vi "Adquisicion.vi"(5 "Stop (F)":bool) -> (20 "Image Out":T1(plugin-control), 26 "Stopped":bool, 27 "error out":errorcluster)   [LabVIEW 2017]
doc: "Creates, and edits acquisitions using the NI Vision Acquisition Express VI.\n\nThe NI Vision Acquisition Wizard is launched by placing the Express VI on the block diagram. Select an acquisition source and configure an acquisition using NI-IMAQ, NI-IMAQdx, or simulate an acquisition by reading an AVI or image files from a folder. After an acquisition is configured, select controls and indicators to be able to programmatically set in LabVIEW. Double-click the Vision Acquisition Express VI to edit the acquisition.\n\nNote: Any images created by the Express VI need to be disposed after use. Use the IMAQ Dispose.vi to cleanup the images output by the Express VI when they are no longer needed."
uses:
  <vilib>/vision/driver/NI_Vision_Acquisition_Software.lvlib
  <vilib>/vision/driver/Vision Acquisition Express Utility VIs.llb/Vision Acquisition Path Convert (String).vi
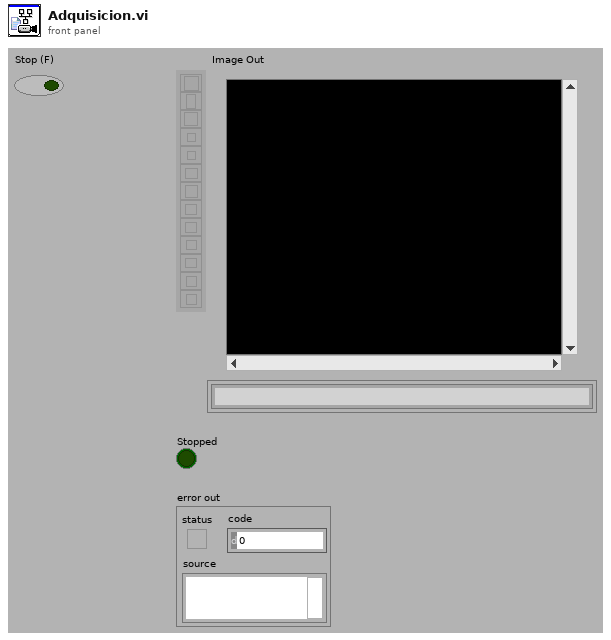
[diagram p1: front panel]
types:
  T1 = typedef "IMAQ Image.ctl" = refnum<image>
  T2 = typedef "IMAQdx.ctl" = refnum<k21>
  T3 = cluster{"File Type":string, "Quality":u32, "Compress":bool, "Lossless":bool, "Ratio":sgl, "Codec":string, "Frame Rate":u32, "Limit Frames":bool, "Max Frames":u32}
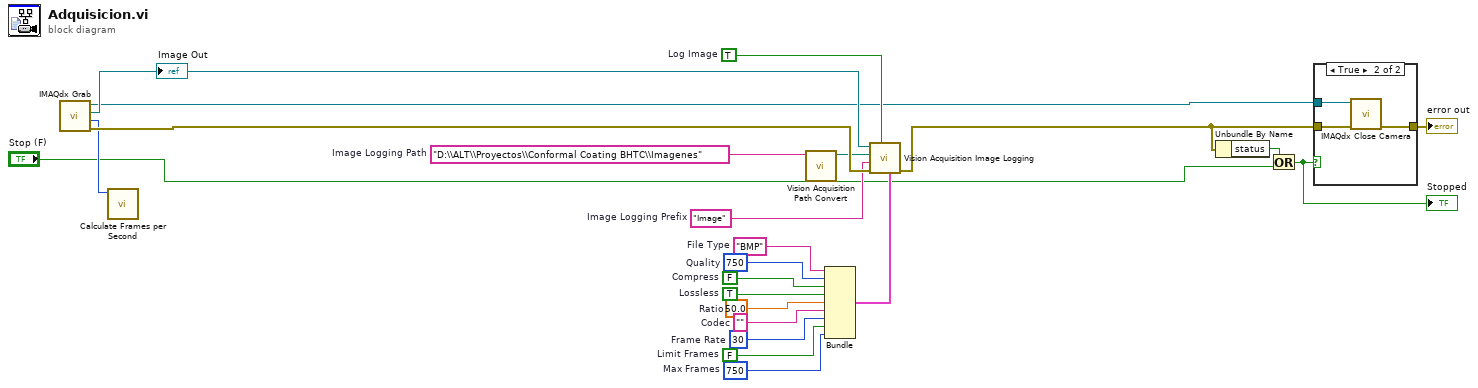
[diagram p0: block diagram]
diagram:
  w6 = "D:\\ALT\\Proyectos\\Conformal Coating BHTC\\Imagenes"  # Image Logging Path
  w9 = TRUE  # Log Image
  w20 = "Image"  # Image Logging Prefix
  w15 = sgl 50.0  # Ratio
  w16 = TRUE  # Lossless
  w17 = FALSE  # Compress
  w18 = u32 750  # Quality
  w14 = ""  # Codec
  w13 = u32 30  # Frame Rate
  w11 = u32 750  # Max Frames
  w12 = FALSE  # Limit Frames
  w19 = "BMP"  # File Type
  n1 = call <vilib>:"IMAQdx Grab.vi"() -> ("error out"=w23:errorcluster, "Buffer Number Out"=w22:u32, "Image Out"=w21:T1, "Session Out"=w5:T2, "error in"=w26:errorcluster, "Image In"=w25:T1, "Session In"=w24:T2)  [unwired: 1 in, 4 out]
  "Image Out" <- w21
  n2 = call <vilib>:"Calculate Frames per Second.vi"("Buffer Number"=w22) -> ()  [unwired: 2 in, 9 out]
  n3 = call-poly <vilib>:"Vision Acquisition Path Convert.vi"("Path In"=w6) -> ("Path Out"=w7:path)  [unwired: 10 in]
  n4 = Bundle("File Type"=w19, "Quality"=w18, "Compress"=w17, "Lossless"=w16, "Ratio"=w15, "Codec"=w14, "Frame Rate"=w13, "Limit Frames"=w12, "Max Frames"=w11) -> (w8:T3)  [unwired: 1 out]
  n5 = call <vilib>:"Vision Acquisition Image Logging.vi"("File Settings"=w8, "Log Image"=w9, "error in (no error)"=w23, "Image Logging Prefix"=w20, "Image Logging Path"=w7, "Image In"=w21) -> ("error out"=w10:errorcluster)  [unwired: 1 in, 4 out]
  n6 = Unbundle By Name(w10) -> ("status"=w1:bool)
  n7 = Or(x=w1, y="Stop (F)") -> (x .or. y?=w2:bool)
  "Stopped" <- w2
  n8 = case "Case Structure_template1" shown="True" w2 {
    tunnel: [w27 w29] -> w4
    tunnel: w10 -> [w27 w30]
    tunnel: w5 -> [_ w28]
    frame False {
    }
    frame True {
      n9 = call <vilib>:"IMAQdx Close Camera.vi"("error in"=w30, "Session In"=w28) -> ("error out"=w29:errorcluster)  [unwired: 9 out]
    }
  }
  "error out" <- w4
